vi "通过布尔数组获取坐标.vi"(0 "数组":bool[][](array[boolean])) -> (1 "X":i32[](array[numeric]), 2 "Y":i32[](array[numeric]))   [LabVIEW 2017]
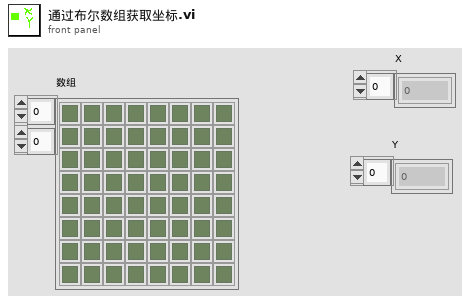
[diagram p1: front panel]
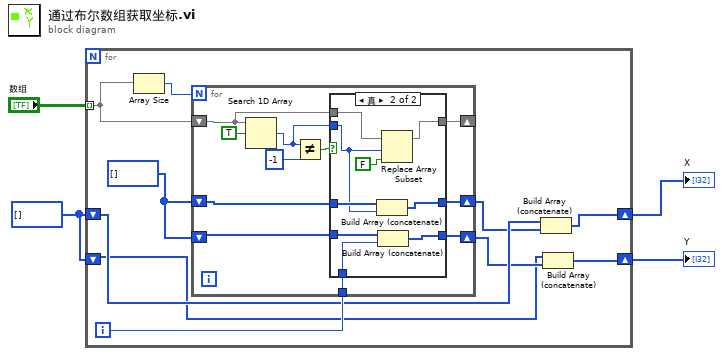
[diagram p0: block diagram]
diagram:
  w3 = i32[] []
  n1 = for {
    tunnel: "数组" -> [w13] mode=indexing
    shift-right: [w6] -> w2
    shift-left: w3 -> [w10]
    shift-right: [w5] -> w1
    shift-left: w3 -> [w7]
    i -> [w12]
    w11 = i32[] []
    n2 = Array Size(array=w13) -> (size(s)=w14:i32)
    n3 = for {
      N: w14 -> [_]
      shift-right: [w20] -> _
      shift-left: w13 -> [w21]
      shift-right: [w18] -> w9
      shift-left: w11 -> [w19]
      shift-right: [w17] -> w8
      shift-left: w11 -> [w16]
      tunnel: w12 -> [w15]
      n4 = Search 1D Array(1D array=w21, element=TRUE ("元素")) -> (index of element=w22:i32)  [unwired: 1 in]
      n5 = Not Equal?(x=w22, y=-1) -> (x != y?=w23:bool)
      n6 = case shown="真" w23 {
        tunnel: w22 -> [_ w30]
        tunnel: w21 -> [w28 w37]
        tunnel: [w28 w35] -> w20
        tunnel: w19 -> [w27 w34]
        tunnel: [w27 w33] -> w18
        tunnel: [w26 w32] -> w17
        tunnel: w16 -> [w26 w31]
        tunnel: w15 -> [_ w29]
        frame False {
        }
        frame True {
          n7 = Build Array (concatenate)(w34, w30) -> (w33:i32[])
          n8 = Build Array (concatenate)(w31, w29) -> (w32:i32[])
          n9 = Replace Array Subset(array=w37, new element=FALSE ("新元素/子数组"), index=w30) -> (w35:bool[])
        }
      }
    }
    n10 = Build Array (concatenate)(w10, w9) -> (w6:i32[])
    n11 = Build Array (concatenate)(w7, w8) -> (w5:i32[])
  }
  "X" <- w2
  "Y" <- w1
